vi "DownloadBulkSBDFiles.vi"(8 "error in (no error)":errorcluster, 10 "Array":T1(array[cluster]), 11 "Value":string) -> (0 "error out":errorcluster)   [LabVIEW 2014]
uses:
  <vilib>/FTP/NI_FTP.lvlib
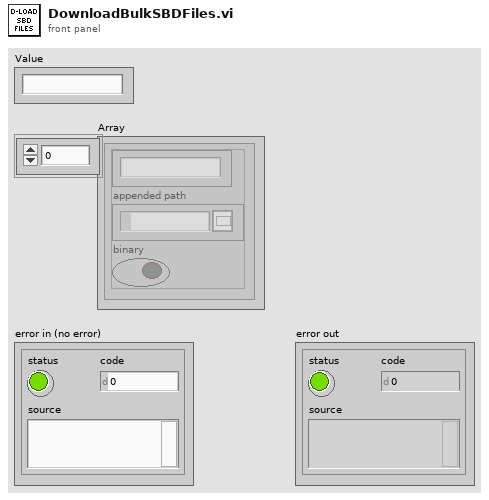
[diagram p1: front panel]
types:
  T1 = cluster{"String":string, "appended path":path, "binary":bool}[]
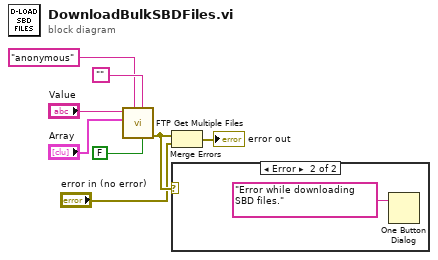
[diagram p0: block diagram]
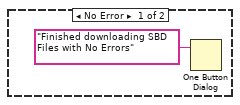
[diagram p2: hidden frame]
diagram:
  n1 = call <vilib>:"FTP Get Multiple Files.vi"("active (T)"=FALSE, "password"="", "user"="anonymous", "file specifications"="Array", "host"="Value") -> ("error out"=w8:errorcluster)  [unwired: 5 in, 1 out]
  n2 = Merge Errors(w8, "error in (no error)") -> (→"error out":errorcluster)
  n3 = case shown="Error" w8 {
    frame No Error {
      n4 = One Button Dialog(message="Finished downloading SBD Files with No Errors") -> ()  [unwired: 1 in, 1 out]
    }
    frame Error {
      n5 = One Button Dialog(message="Error while downloading SBD files.") -> ()  [unwired: 1 in, 1 out]
    }
  }
